vi "MTM2_logEvent_m2AssemblyInPosition.vi"(8 "error in (no error)":errorcluster, 11 "logevent_m2AssemblyInPosition_Ctl":T1) -> (0 "error out":errorcluster, 2 "function return":i32, 3 "logevent_m2AssemblyInPosition_Ctl out":T1)   [LabVIEW 2018, in "SALLV_MTM2.lvlib"]
doc: "int MTM2_shm_logEvent_m2AssemblyInPositionLV(MTM2_logevent_m2AssemblyInPositionLV *logevent_m2AssemblyInPosition_Ctl );"
uses:
  DataTypes/logevent_m2AssemblyInPosition.ctl
  SALLV_MTM2.lvlib
  SALLV_MTM2.so
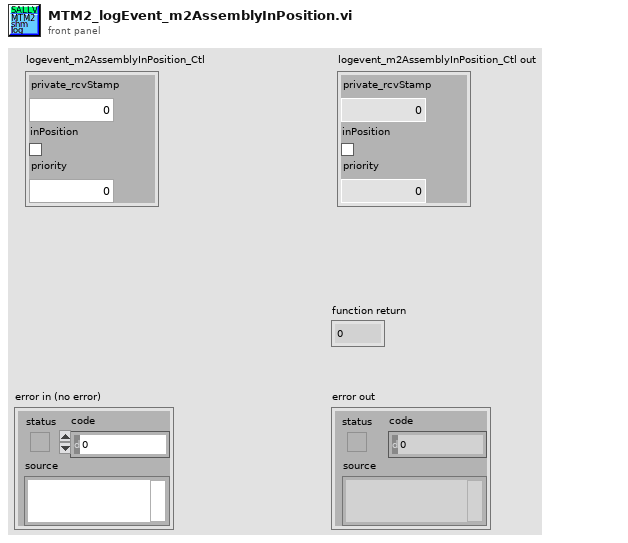
[diagram p1: front panel]
types:
  T1 = typedef "SALLV_MTM2.lvlib/logevent_m2AssemblyInPosition.ctl" = cluster{"private_rcvStamp":dbl, "inPosition":bool, "priority":i32}
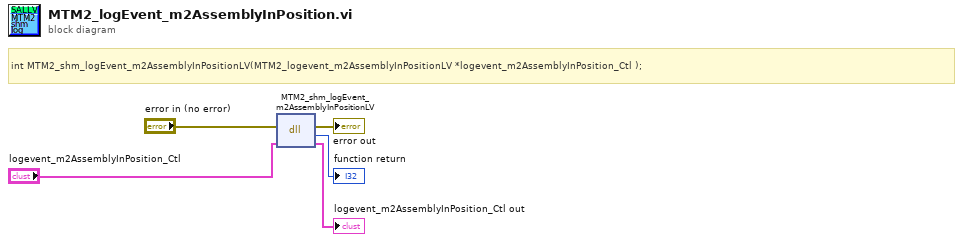
[diagram p0: block diagram]
diagram:
  # "int MTM2_shm_logEvent_m2AssemblyInPositionLV(MTM2_logevent_m2AssemblyInPositionLV *logevent_m2AssemblyInPosition_Ctl );"
  n1 = dll-call lib="home/ttsai/Documents/salTestLabViewApi/SALLV_MTM2/SALLV_MTM2.*" fn="MTM2_shm_logEvent_m2AssemblyInPositionLV"(error in="error in (no error)", "logevent_m2AssemblyInPosition_Ctl"="logevent_m2AssemblyInPosition_Ctl") -> (error out=→"error out":errorcluster, →"function return":i32, "logevent_m2AssemblyInPosition_Ctl"=→"logevent_m2AssemblyInPosition_Ctl out":T1)  [unwired: 2 in, 1 out]
